vi "Invoke RT VI.vi"(6 "Run Time":u32, 8 "error in (no error)":errorcluster, 9 "configuration file path":path, 10 "target alias":string, 11 "reference":refnum<vi>) -> (0 "error out":errorcluster, 1 "engine status":string, 2 "invoked VI error out":errorcluster, 3 "reference out":refnum<vi>)   [LabVIEW 2014]
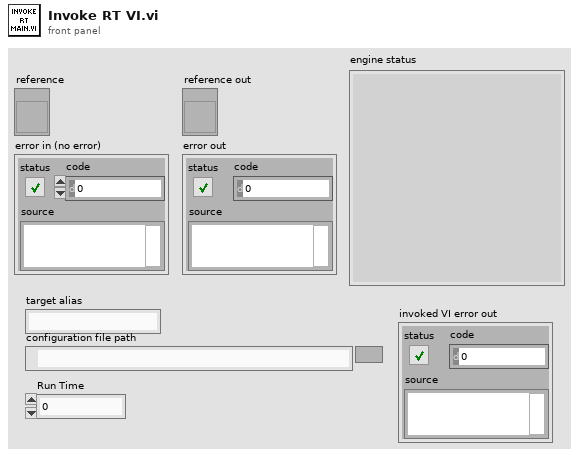
[diagram p1: front panel]
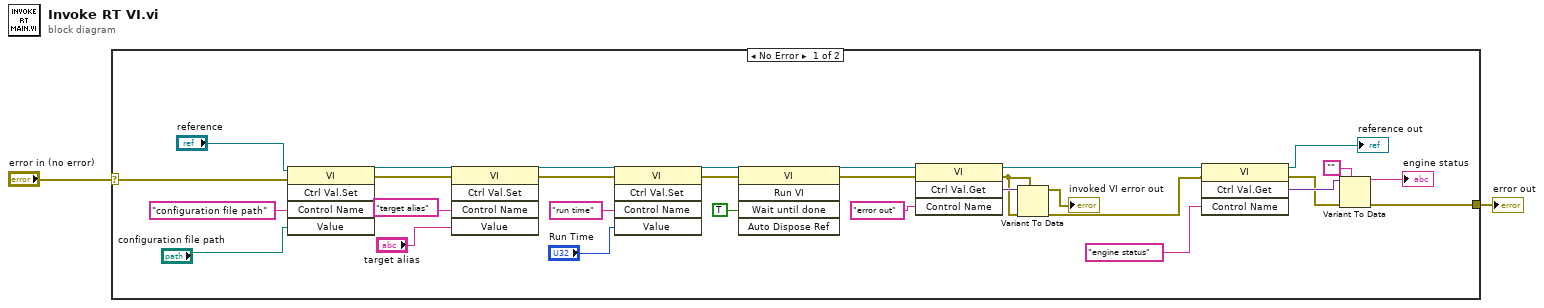
[diagram p0: block diagram]
diagram:
  n1 = case shown="No Error" "error in (no error)" {
    selector: "error in (no error)" -> [w13 w33]
    tunnel: [w3 w33] -> w2
    frame No Error {
      n2 = invoke class="VI" method="Ctrl Val.Set"(reference="reference", error in=w13, "Control Name"="configuration file path", "Value"="configuration file path") -> (reference out=w15:refnum<vi>, error out=w21:errorcluster)  [unwired: 1 in, 3 out]
      n3 = invoke class="VI" method="Ctrl Val.Set"(reference=w15, error in=w21, "Control Name"="target alias", "Value"="target alias") -> (reference out=w24:refnum<vi>, error out=w23:errorcluster)  [unwired: 1 in, 3 out]
      n4 = invoke class="VI" method="Ctrl Val.Set"(reference=w24, error in=w23, "Control Name"="run time", "Value"="Run Time") -> (reference out=w26:refnum<vi>, error out=w27:errorcluster)  [unwired: 1 in, 3 out]
      n5 = invoke class="VI" method="Run VI"(reference=w26, error in=w27, "Wait until done"=TRUE ("Wait Until Done")) -> (reference out=w28:refnum<vi>, error out=w31:errorcluster)  [unwired: 2 in, 3 out]
      n6 = invoke class="VI" method="Ctrl Val.Get"(reference=w28, error in=w31, "Control Name"="error out") -> (reference out=w12:refnum<vi>, error out=w11:errorcluster, "Get Control Value Variant"=w30:variant)  [unwired: 1 in, 1 out]
      n7 = Variant To Data(error in=w11, type=w11, Variant=w30) -> (data=→"invoked VI error out":errorcluster, error out=w10:errorcluster)
      n8 = invoke class="VI" method="Ctrl Val.Get"(reference=w12, error in=w10, "Control Name"="engine status") -> (reference out=→"reference out":refnum<vi>, error out=w4:errorcluster, "Get Control Value Variant"=w5:variant)  [unwired: 1 in, 1 out]
      n9 = Variant To Data(error in=w4, type="", Variant=w5) -> (data=→"engine status":string, error out=w3:errorcluster)
    }
    frame Error {
    }
  }
  "error out" <- w2
